vi "CreateRegistryFile.vi"() -> ()   [LabVIEW 2014]
uses:
  <vilib>/Utility/file.llb/Read From Spreadsheet File (string).vi
panel:
  in  "Stop":bool
  in  "Run":bool
  # "Create Variation Registry File"
  # "This application creates a TDMS file that is used to store version numbers\nof all the executables in the HIL setup.\n\nIf the TDMS file has already been created, avoid running this application. Run Register Change, instead.\n\nTo run this application, you need a txt file, in which you have name all \nexecutables (or any other components) that are in the test environment.\nEach name shall be written in one row."
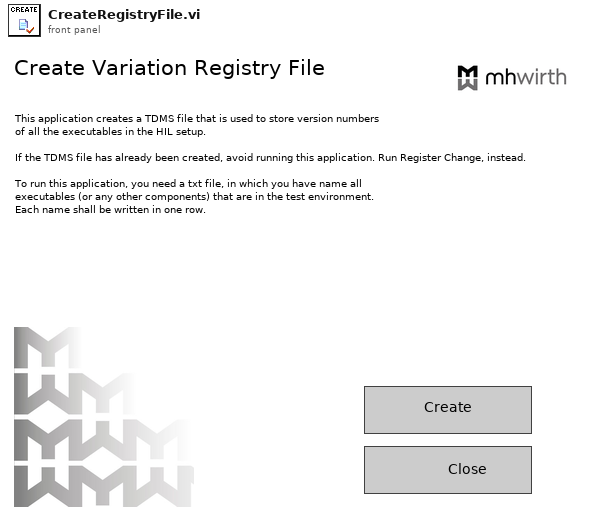
[diagram p1: front panel]
types:
  T1 = enum32{"invalid app kind", "Development System", "Run Time System", "Student Edition", "Embedded LabVIEW", "Evaluation", "Custom"}
  T2 = enum16{"open", "open or create", "create or replace", "create", "open (read-only)"}
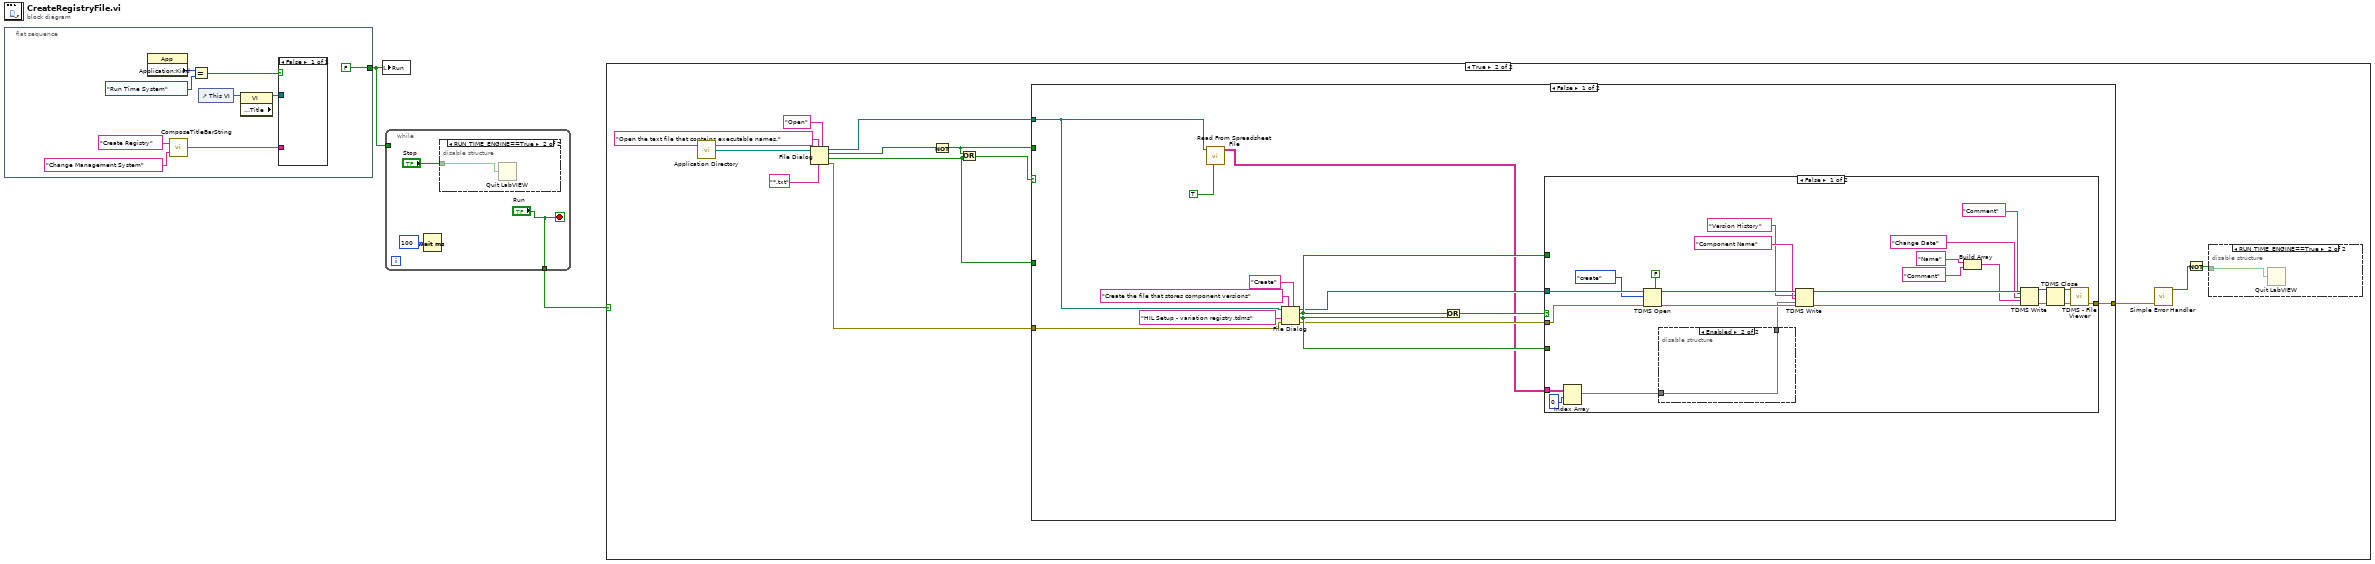
[diagram p0: block diagram]
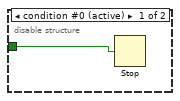
[diagram p2: hidden frame]
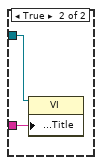
[diagram p3: hidden frame]
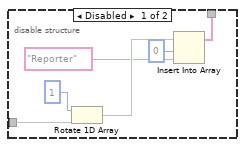
[diagram p6: hidden frame]
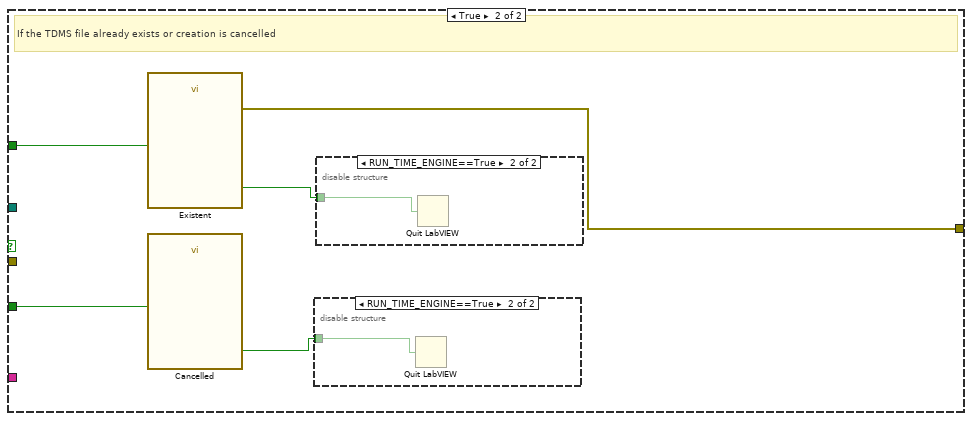
[diagram p7: hidden frame]
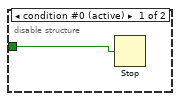
[diagram p8: hidden frame]
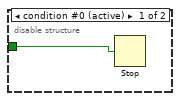
[diagram p9: hidden frame]
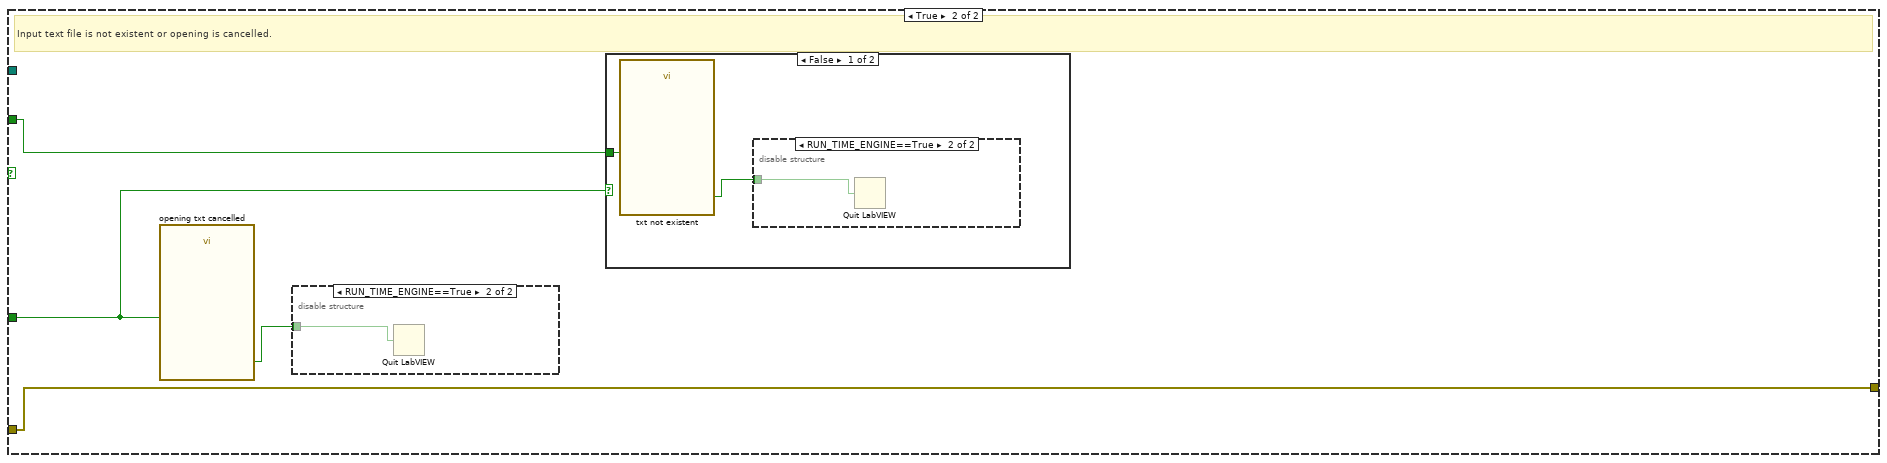
[diagram p10: hidden frame]
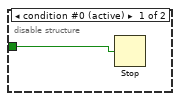
[diagram p11: hidden frame]
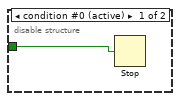
[diagram p13: hidden frame]
diagram:
  n1 = flat-sequence {
    tunnel: [FALSE ("Run")] -> w1
    frame #0 {
      n2 = property on="Property Node" class="App"() -> ("Application:Kind"=w8:T1)  [unwired: 2 in, 2 out]
      n3 = call "ComposeTitleBarString.vi"("ProjectName"="Change Management System" ("Application"), "Application"="Create Registry") -> ("TitleBar"=w10:string)
      n4 = Equal?(x=w8, y=T1."Run Time System" ("Applikation:Typ")) -> (x = y?=w9:bool)
      n5 = control-ref of="This VI"() -> (w6:refnum<vi>)
      n6 = property on="Property Node" class="VI" props=["Front Panel.Title"](reference=w6) -> (reference out=w5:refnum<vi>)  [unwired: 1 in, 2 out]
      n7 = case shown="False" w9 {
        tunnel: w10 -> [_ w13]
        tunnel: w5 -> [_ w12]
        frame False {
        }
        frame True {
          n8 = property class="VI"(reference=w12, "Front Panel.Title"=w13) -> ()  [unwired: 1 in, 2 out]
        }
      }
    }
  }
  n9 = local write "Run"(w1) -> ()
  n10 = while {
    tunnel: ["Run"] -> w2
    tunnel: w1 -> [_]
    stop <- "Run" stop-if-true
    n11 = Wait (ms)(milliseconds to wait=u32 100) -> ()  [unwired: 1 out]
    n12 = disable-structure shown="RUN_TIME_ENGINE==True" {
      disable-tunnel: "Stop" -> [w17 w18]
      frame condition #0 (active) {
        n13 = Stop(stop? (T)=w17) -> ()
      }
      frame condition #1 {
        n14 = Quit LabVIEW(quit? (T)=w18) -> ()
      }
    }
  }
  n15 = case shown="True" w2 {
    frame False {
    }
    frame True {
      n16 = call <vilib>:"Application Directory.vi"() -> ("Application Directory"=w19:path)
      n17 = File Dialog(5:"Open" ("button label"), 6:"*.txt" ("default name"), 7:"Open the text file that contains executable names." ("prompt"), 11:w19) -> (0:w24:errorcluster, 1:w25:bool, 2:w28:bool, 3:w22:path)  [unwired: 2 in, 1 out]
      n18 = Not(x=w28) -> (.not. x?=w26:bool)
      n19 = Or(x=w26, y=w25) -> (x .or. y?=w27:bool)
      n20 = case shown="False" w27 {
        tunnel: w26 -> [_ w89]
        tunnel: w25 -> [_ w86]
        tunnel: w24 -> [w37 w87]
        tunnel: [w36 w87] -> w23
        tunnel: w22 -> [w33 _]
        frame False {
          n21 = call-poly <vilib>:"Read From Spreadsheet File.vi"("transpose (no:F)"=TRUE, "file path (dialog if empty)"=w33) -> ("all rows"=w35:string[][])  [unwired: 5 in, 4 out]
          n22 = File Dialog(5:"Create" ("button label"), 7:"Create the file that stores component versions" ("prompt"), 8:w37, 9:"HIL Setup - variation registry.tdms" ("default name"), 11:w33) -> (0:w42:errorcluster, 1:w43:bool, 2:w44:bool, 3:w41:path)  [unwired: 2 out]
          n23 = Or(x=w44, y=w43) -> (x .or. y?=w45:bool)
          n24 = case shown="False" w45 {
            tunnel: w44 -> [_ w81]
            tunnel: w43 -> [_ w80]
            tunnel: w42 -> [w68 _]
            tunnel: w41 -> [w69 _]
            tunnel: [w59 w79] -> w36
            tunnel: w35 -> [w49 _]
            frame False {
              n25 = Index Array(array=w49, index (row)=0 ("disabled index (col)")) -> (element=w48:string[])  [unwired: 1 in]
              n26 = TDMS Open(5:FALSE ("create index file? (T)"), 8:w68, 10:T2."create" ("operation (0:open)"), 11:w69) -> (0:w65:errorcluster, 3:w64:refnum<k34>)  [unwired: 3 in]
              n27 = disable-structure shown="Enabled" {
                disable-tunnel: w48 -> [w74 w76]
                disable-tunnel: [w70 w76] -> w47
                frame Disabled {
                  n28 = Rotate 1D Array(1:w74, 2:1 ("n")) -> (0:w73:string[])
                  n29 = Insert Into Array(array=w73, index=0, new element="Reporter" ("new element/subarray")) -> (w70:string[])
                }
                frame Enabled {
                }
              }
              n30 = TDMS Write(0:w64, 5:"Version History" ("group name in (Untitled)"), 7:"Component Name" ("group name in (Untitled)"), 9:w47, 11:w65) -> (4:w54:refnum<k34>, 15:w53:errorcluster)  [unwired: 1 in, 2 out]
              n31 = Build Array("Name" ("group name in (Untitled)"), "Comment" ("group name in (Untitled)")) -> (w51:string[])
              n32 = TDMS Write(0:w54, 5:"Comment" ("group name in (Untitled)"), 7:"Change Date" ("group name in (Untitled)"), 9:w51, 11:w53) -> (4:w56:refnum<k34>, 15:w55:errorcluster)  [unwired: 1 in, 2 out]
              n33 = TDMS Close(8:w55, 11:w56) -> (0:w61:errorcluster, 3:w60:path)
              n34 = call <vilib>:"TDMS - File Viewer.vi"("error in (no error)"=w61, "file path"=w60) -> ("error out"=w59:errorcluster)  [unwired: 4 in, 1 out]
            }
            frame True {
              # "If the TDMS file already exists or creation is cancelled"
              n35 = call "Existent"("Enable"=w81) -> ("error out"=w79:errorcluster, "OK"=w77:bool)  [unwired: 9 in]
              n36 = call "Cancelled"("Enable"=w80) -> ("OK"=w78:bool)  [unwired: 9 in, 1 out]
              n37 = disable-structure shown="RUN_TIME_ENGINE==True" {
                disable-tunnel: w78 -> [w84 w85]
                frame condition #0 (active) {
                  n38 = Stop(stop? (T)=w84) -> ()
                }
                frame condition #1 {
                  n39 = Quit LabVIEW(quit? (T)=w85) -> ()
                }
              }
              n40 = disable-structure shown="RUN_TIME_ENGINE==True" {
                disable-tunnel: w77 -> [w82 w83]
                frame condition #0 (active) {
                  n41 = Stop(stop? (T)=w82) -> ()
                }
                frame condition #1 {
                  n42 = Quit LabVIEW(quit? (T)=w83) -> ()
                }
              }
            }
          }
        }
        frame True {
          # "Input text file is not existent or opening is cancelled."
          n43 = call "opening txt cancelled"("Enable"=w86) -> ("OK"=w88:bool)  [unwired: 9 in, 1 out]
          n44 = disable-structure shown="RUN_TIME_ENGINE==True" {
            disable-tunnel: w88 -> [w94 w95]
            frame condition #0 (active) {
              n45 = Stop(stop? (T)=w94) -> ()
            }
            frame condition #1 {
              n46 = Quit LabVIEW(quit? (T)=w95) -> ()
            }
          }
          n47 = case shown="False" w86 {
            tunnel: w89 -> [w91 _]
            frame False {
              n48 = call "txt not existent"("Enable"=w91) -> ("OK"=w90:bool)  [unwired: 9 in, 1 out]
              n49 = disable-structure shown="RUN_TIME_ENGINE==True" {
                disable-tunnel: w90 -> [w92 w93]
                frame condition #0 (active) {
                  n50 = Stop(stop? (T)=w92) -> ()
                }
                frame condition #1 {
                  n51 = Quit LabVIEW(quit? (T)=w93) -> ()
                }
              }
            }
            frame True {
            }
          }
        }
      }
      n52 = call <vilib>:"Simple Error Handler.vi"("error in (no error)"=w23) -> ("error?"=w20:bool)  [unwired: 4 in, 4 out]
      n53 = Not(x=w20) -> (.not. x?=w21:bool)
      n54 = disable-structure shown="RUN_TIME_ENGINE==True" {
        disable-tunnel: w21 -> [_ w32]
        frame condition #0 (active) {
        }
        frame condition #1 {
          n55 = Quit LabVIEW(quit? (T)=w32) -> ()
        }
      }
    }
  }
